vi "Make ear folder.vi"(3 "Error bundle in.":errorcluster, 4 "Ear folder number.":dbl format="%.2f", 5 "Date folder path name.":path, 6 "Date folder path name (string).":string) -> (0 "Error bundle out.":errorcluster, 1 "Ear folder path name.":path, 2 "Ear folder path name (string).":string)   [LabVIEW 2010]
panel:
  out "?":dbl format="%.2f"
  # "Inputs:"
  # "Outputs:"
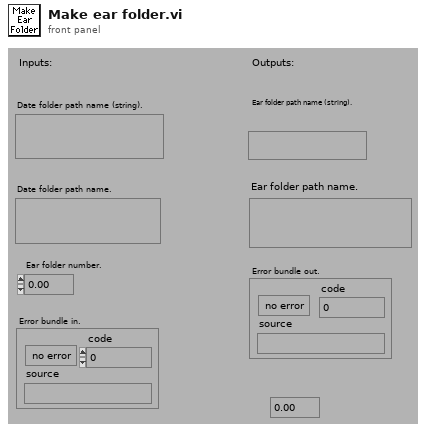
[diagram p1: front panel]
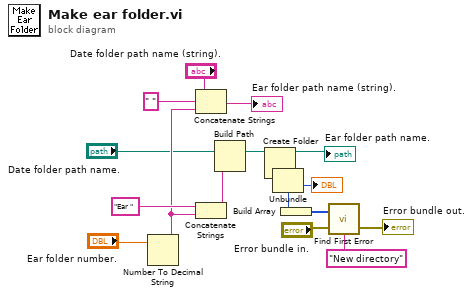
[diagram p0: block diagram]
diagram:
  n1 = Number To Decimal String(number="Ear folder number.") -> (decimal integer string=w12:string)  [unwired: 1 out]
  n2 = Concatenate Strings("Date folder path name (string).", " ", w12) -> (→"Ear folder path name (string).":string)
  n3 = Concatenate Strings("Ear ", w12) -> (w15:string)
  n4 = Build Path(base path="Date folder path name.", name or relative path=w15) -> (appended path=w16:path)
  n5 = Create Folder(path (use dialog)=w16) -> (created path=→"Ear folder path name.":path, error out=w2:errorcluster)  [unwired: 1 in, 2 out]
  n6 = Unbundle(w2) -> ("code"=w1:i32)  [unwired: 2 out]
  "?" <- w1
  n7 = Build Array(w1) -> (w7:i32[])
  n8 = call <vilib>:"Find First Error.vi"("error in (no error)"="Error bundle in.", "source messages"="New directory", "error codes"=w7) -> ("error out"=→"Error bundle out.":errorcluster)  [unwired: 2 out]
